vi "check for event.vi"(11 "event queue in":T2) -> (1 "empty?":bool, 2 "event":T1, 3 "event queue out":T2)   [LabVIEW 2013, in "data bus events.lvlib"]
uses:
  data bus events.lvlib
  event queue.ctl
  event.ctl
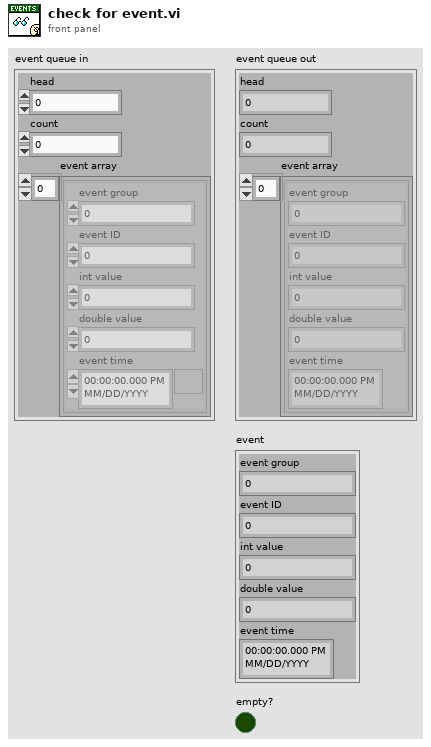
[diagram p1: front panel]
types:
  T1 = typedef "data bus events.lvlib/event.ctl" = cluster{"event group":i64, "event ID":i64, "int value":i64, "double value":dbl, "event time":timestamp}
  T2 = typedef "data bus events.lvlib/event queue.ctl" = cluster{"head":i32, "count":i32, "event array":T1[]}
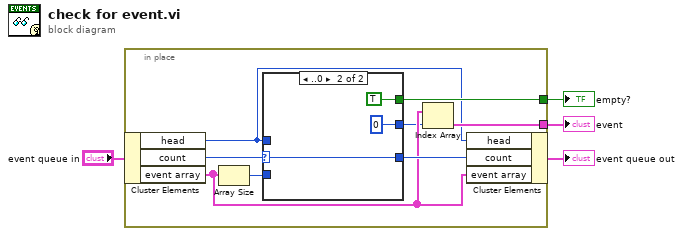
[diagram p0: block diagram]
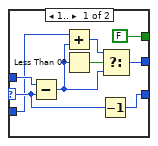
[diagram p2: hidden frame]
diagram:
  n1 = in-place {
    in-place-border: [w11] -> w4
    in-place-border: [w9] -> w3
    n2 = in-place-cluster #1("event queue in") -> ("head"=w6:i32, "count"=w12:i32, "event array"=w8:T1[])
    n3 = Array Size(array=w8) -> (size(s)=w7:i32)
    n4 = case shown="..0" w12 {
      selector: w12 -> [w18 w23]
      tunnel: w6 -> [w19 _]
      tunnel: [FALSE TRUE] -> w11
      tunnel: [w21 w23] -> w10
      tunnel: w7 -> [w16 _]
      tunnel: [w13 0] -> w5
      frame 1.. {
        n5 = Subtract(x=w19, y=w18) -> (x-y=w14:i32)
        n6 = Add(x=w16, y=w14) -> (x+y=w15:i32)
        n7 = Less Than 0?(x=w14) -> (x < 0?=w17:bool)
        n8 = Decrement(x=w18) -> (x-1=w21:i32)
        n9 = Select(t=w15, s=w17, f=w14) -> (s? t:f=w13:i32)
      }
      frame ..0 {
      }
    }
    n10 = Index Array(array=w8, index=w5) -> (element=w9:T1)
    n11 = in-place-cluster #1("head"=w6, "count"=w10, "event array"=w8) -> (→"event queue out":T2)
  }
  "empty?" <- w4
  "event" <- w3
